vi "TSCAN_LoadCANDBC.vi"(7 "AIdIn":u32, 8 "错误输入（无错误）":errorcluster, 9 "ABindChannels":i32[](array[ring])=[0] items=["CHN1", "CHN2", "CHN3", "CHN4", "CHN5", "CHN6", "CHN7", "CHN8", "CHN9", "CHN10", "CHN11", "CHN12", "CHN13", "CHN14", "CHN15", "CHN16", "CHN17", "CHN18", "CHN19", "CHN20", "CHN21", "CHN22", "CHN23", "CHN24", "CHN25", "CHN26", "CHN27", "CHN28", "CHN29", "CHN30", "CHN31", "CHN32"], 10 "ADBCAbsolutePath":path=path "C:/Users/DYR/Desktop/M110.dbc", 11 "路径输入":path) -> (0 "错误输出":errorcluster, 1 "AIdOut":u32, 3 "路径输出":path, 4 "x = 0?":bool)   [LabVIEW 2019]
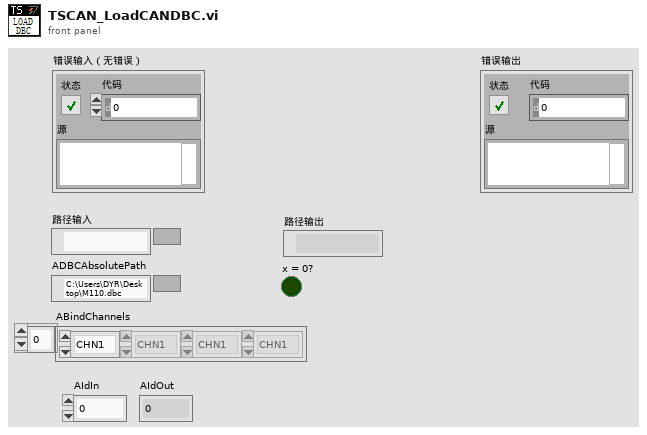
[diagram p1: front panel]
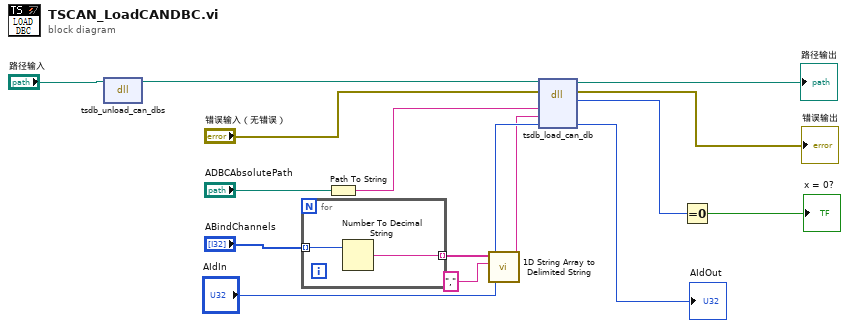
[diagram p0: block diagram]
diagram:
  n1 = dll-call lib="PTH27abs EDemo同星\nTSCAN_V1.0ConfigTSMaster.dll" fn="tsdb_unload_can_dbs"(path in="路径输入") -> (path out=w1:path)  [unwired: 3 in, 1 out]
  n2 = for {
    tunnel: "ABindChannels" -> [w17] mode=indexing
    tunnel: [w16] -> w5 mode=indexing
    n3 = Number To Decimal String(number=w17) -> (decimal integer string=w16:string)  [unwired: 1 in]
  }
  n4 = Path To String(path="ADBCAbsolutePath") -> (string=w13:string)
  n5 = call <vilib>:"1D String Array to Delimited String.vi"("delimiter"=",", "string array"=w5) -> ("delimited string"=w3:string)  [unwired: 9 in]
  n6 = dll-call lib="PTH27abs EDemo同星\nTSCAN_V1.0ConfigTSMaster.dll" fn="tsdb_load_can_db"(path in=w1, error in="错误输入（无错误）", "ADBCAbsolutePath"=w13, "ABindChannels"=w3, "AId"="AIdIn") -> (path out=→"路径输出":path, error out=→"错误输出":errorcluster, "tsdb_load_can_db"=w12:i32, "AId"=→"AIdOut":i32)  [unwired: 3 in]
  n7 = Equal To 0?(x=w12) -> (x = 0?=→"x = 0?":bool)
